vi "Get.vi"(8 "error in (no error)":errorcluster, 11 "MicronMessage in":refnum<class "GRPCMessage.lvclass">) -> (0 "error out":errorcluster, 1 "Payload":string, 2 "Command":string, 3 "MicronMessage out":refnum<class "GRPCMessage.lvclass">)   [LabVIEW 2019, in "MicronGRPCServer.lvlib" / "GRPCMessage.lvclass"]
uses:
  GRPCMessage.lvclass
  GRPCMessage.lvclass/GRPCMessage.ctl
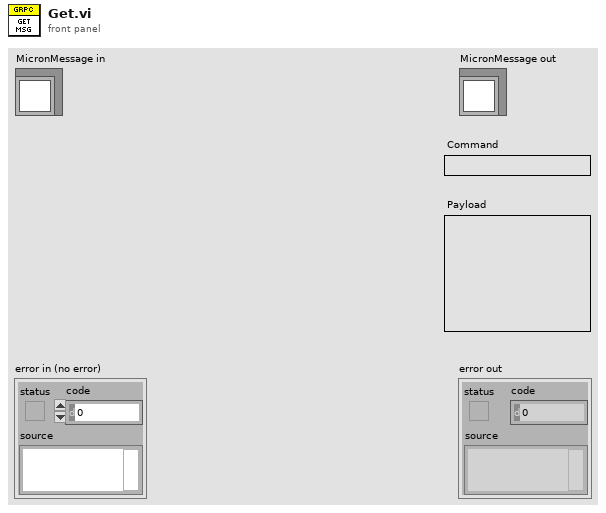
[diagram p1: front panel]
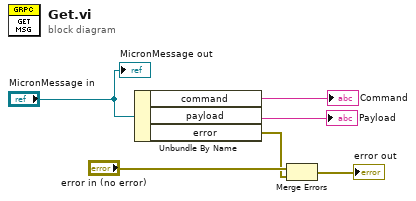
[diagram p0: block diagram]
diagram:
  n1 = Unbundle By Name("MicronMessage in") -> ("command"=→"Command":string, "payload"=→"Payload":string, "error"=w1:errorcluster)
  n2 = Merge Errors("error in (no error)", w1) -> (→"error out":errorcluster)
  "MicronMessage out" <- "MicronMessage in"
